vi "Check Shared Library Version.vi"(8 "error in":errorcluster) -> (0 "error out":errorcluster)   [LabVIEW 2024, in "serenial.io-ase.lvlib" / "ase.lvclass"]
doc: "Checks the version reported by the shared library matches that expected by the LabVIEW library"
uses:
  ase.lvclass
  ase.lvclass/ase.ctl
  serenial.io-ase.32.dll
panel:
  out "Version":string
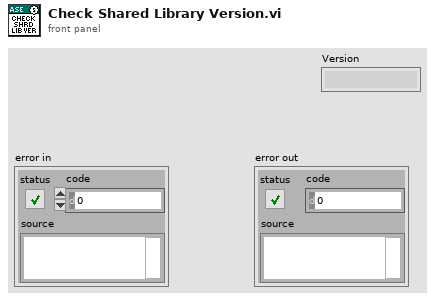
[diagram p1: front panel]
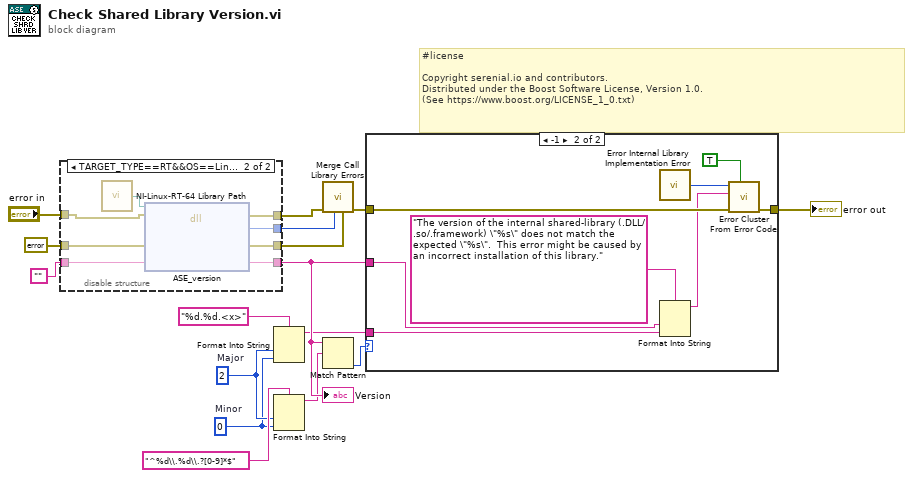
[diagram p0: block diagram]
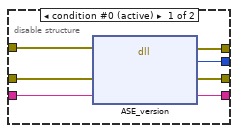
[diagram p2: hidden frame]
diagram:
  w4 = 2  # Major
  w3 = 0  # Minor
  # "#license\n\nCopyright serenial.io and contributors.\nDistributed under the Boost Software License, Version 1.0.\n(See https://www.boost.org/LICENSE_1_0.txt)"
  n1 = disable-structure "Conditional Disable Structure" shown="TARGET_TYPE==RT&&OS==Linux" {
    disable-tunnel: "error in" -> [w23 w31]
    disable-tunnel: [w22 w28] -> w9
    disable-tunnel: [w21 w30] -> w14
    disable-tunnel: [w20 w29] -> w13
    disable-tunnel: [w19 w27] -> w12
    disable-tunnel: errorcluster {"status"=FALSE, "code"=0, "source"=""} ("Library Call Returned Error") -> [w18 w26]
    disable-tunnel: "" ("Version") -> [w17 w25]
    frame condition #0 (active) {
      n2 = dll-call lib="C:/Users/marc/code/sift-streaming/labview/Sift/Dependencies/asynchronous-system-exec-v2.0.0/serenial.io-ase/ase/serenial.io-ase.*.*" fn="ASE_version" ("AsyncSystemExec*.*:wrapperVersion")(error in=w23, "Error Out"=w18, "Version"=w17) -> (error out=w21:errorcluster, "Error Code"=w20:i32, "Error Out"=w19:errorcluster, "Version"=w22:string)  [unwired: 2 in, 1 out]
    }
    frame condition #1 {
      n3 = call "NI-Linux-RT-64 Library Path.vi"() -> ("Path"=w24:path)
      n4 = dll-call lib="?" fn="ASE_version" ("AsyncSystemExec*.*:wrapperVersion")(path in=w24, error in=w31, "Error Out"=w26, "Version"=w25) -> (error out=w30:errorcluster, "Error Code"=w29:i32, "Error Out"=w27:errorcluster, "Version"=w28:string)  [unwired: 1 in, 1 out]
    }
  }
  "Version" <- w9
  n5 = Format Into String(format string="%d.%d.<x>", w4, w3) -> (resulting string=w1:string)  [unwired: 2 in, 1 out]
  n6 = Format Into String(format string="^%d\\.%d\\.?[0-9]*$", w4, w3) -> (resulting string=w5:string)  [unwired: 2 in, 1 out]
  n7 = call "Merge Call Library Errors.vi"("Library Call Returned Error"=w12, "Error Code"=w13, "error in"=w14) -> ("error IO"=w7:errorcluster)  [unwired: 8 in]
  n8 = Match Pattern(string=w9, regular expression=w5) -> (offset past match=w8:i32)  [unwired: 1 in, 3 out]
  n9 = case shown="-1" w8 {
    tunnel: w9 -> [_ w39]
    tunnel: w7 -> [w32 w37]
    tunnel: [w32 w38] -> w16
    tunnel: w1 -> [_ w33]
    frame Default {
    }
    frame -1 {
      n10 = call "Error Internal Library Implementation Error.vi"() -> ("Error Code"=w34:i32)
      n11 = Format Into String(format string="The version of the internal shared-library (.DLL/.so/.framework) \"%s\" does not match the expected \"%s\".  This error might be caused by an incorrect installation of this library.", w39, w33) -> (resulting string=w36:string)  [unwired: 2 in, 1 out]
      n12 = call <vilib>:"Error Cluster From Error Code.vi"("show call chain? (False)"=TRUE, "error in (no error)"=w37, "error message (\"\")"=w36, "error code (0)"=w34) -> ("error out"=w38:errorcluster)  [unwired: 5 in]
    }
  }
  "error out" <- w16
